vi "_Main_ByRuns_DAC2022_V1.0.2.vi"() -> ()   [LabVIEW 2017]
uses:
  <vilib>/Instr/_visa.llb/VISA Configure Serial Port (Instr).vi
panel:
  in  "Bias, kV/cm":dbl
  out "Field, kV/cm":dbl
  out "Current, mA":dbl
  out "Voltage, V":dbl
  in  "COM DAC":refnum<visa-resource-name>
  in  "WaveForm":i32(listbox)
  in  "Auto\nturn OFF":bool=TRUE
  in  "Content":i32(listbox)
  out "LastTrigTimer, s":dbl
  in  "Graph every, cycle":dbl=10.0 min=1.0 max=100.0
  in  "SendPeriod, ms":dbl=100.0 min=10.0 max=10000.0
  out "RunsNeed":i32
  out "Time LOG":cluster{dbl[], dbl[]}(graph)
  out "TrigTimer, s":dbl
  out "Bytes at Port":u32
  out "RecTry":i32
  out "OutVoltage, V":dbl
  in  "Exposition, s":dbl=3.0
  out "Channel 2, V":dbl format="%#_5g"
  out "Channel 1, V":dbl format="%#_5g"
  in  "Stop Button":bool
  in  "Start Button":bool
  in  "Sample H, um":dbl=32.0
  out "VoltageArray, V":dbl[](array[numeric])
  out "Shutter Red":bool
  out "Shutter Green":bool
  in  "Frames In Run":u32=180
  out "Global Frame Done":u32
  out "Now is Run #":u32
  out "Frame In Run Done":u32
  in  "Step, kV/cm":dbl=1.0 min=0.01 max=1000.0
  in  "Amplitude, kV/cm":dbl=10.0 min=10.0 max=1500.0
  in  "LOG file":path
  in  "COM ADC":refnum<visa-resource-name>
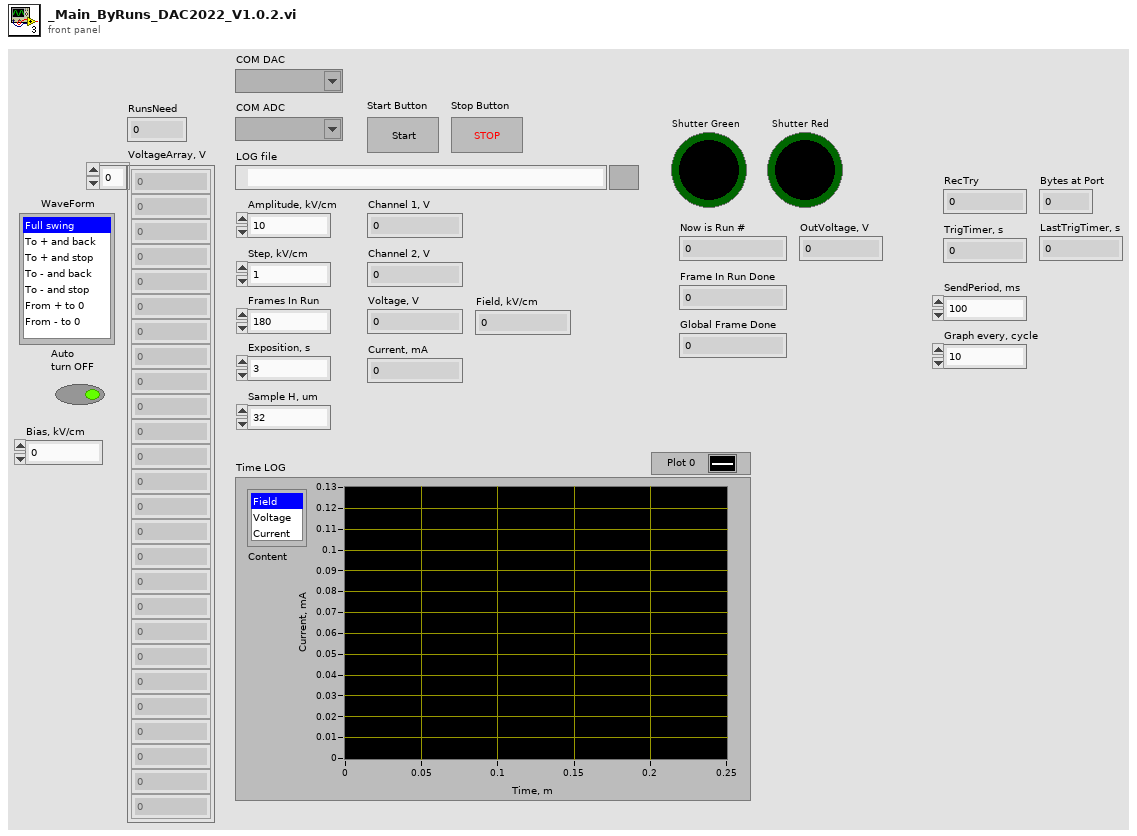
[diagram p1: front panel]
types:
  T1 = cluster{i32, i32, u32, "TrigState":bool, "TrigTimer, s":dbl, "CurrentError":bool}
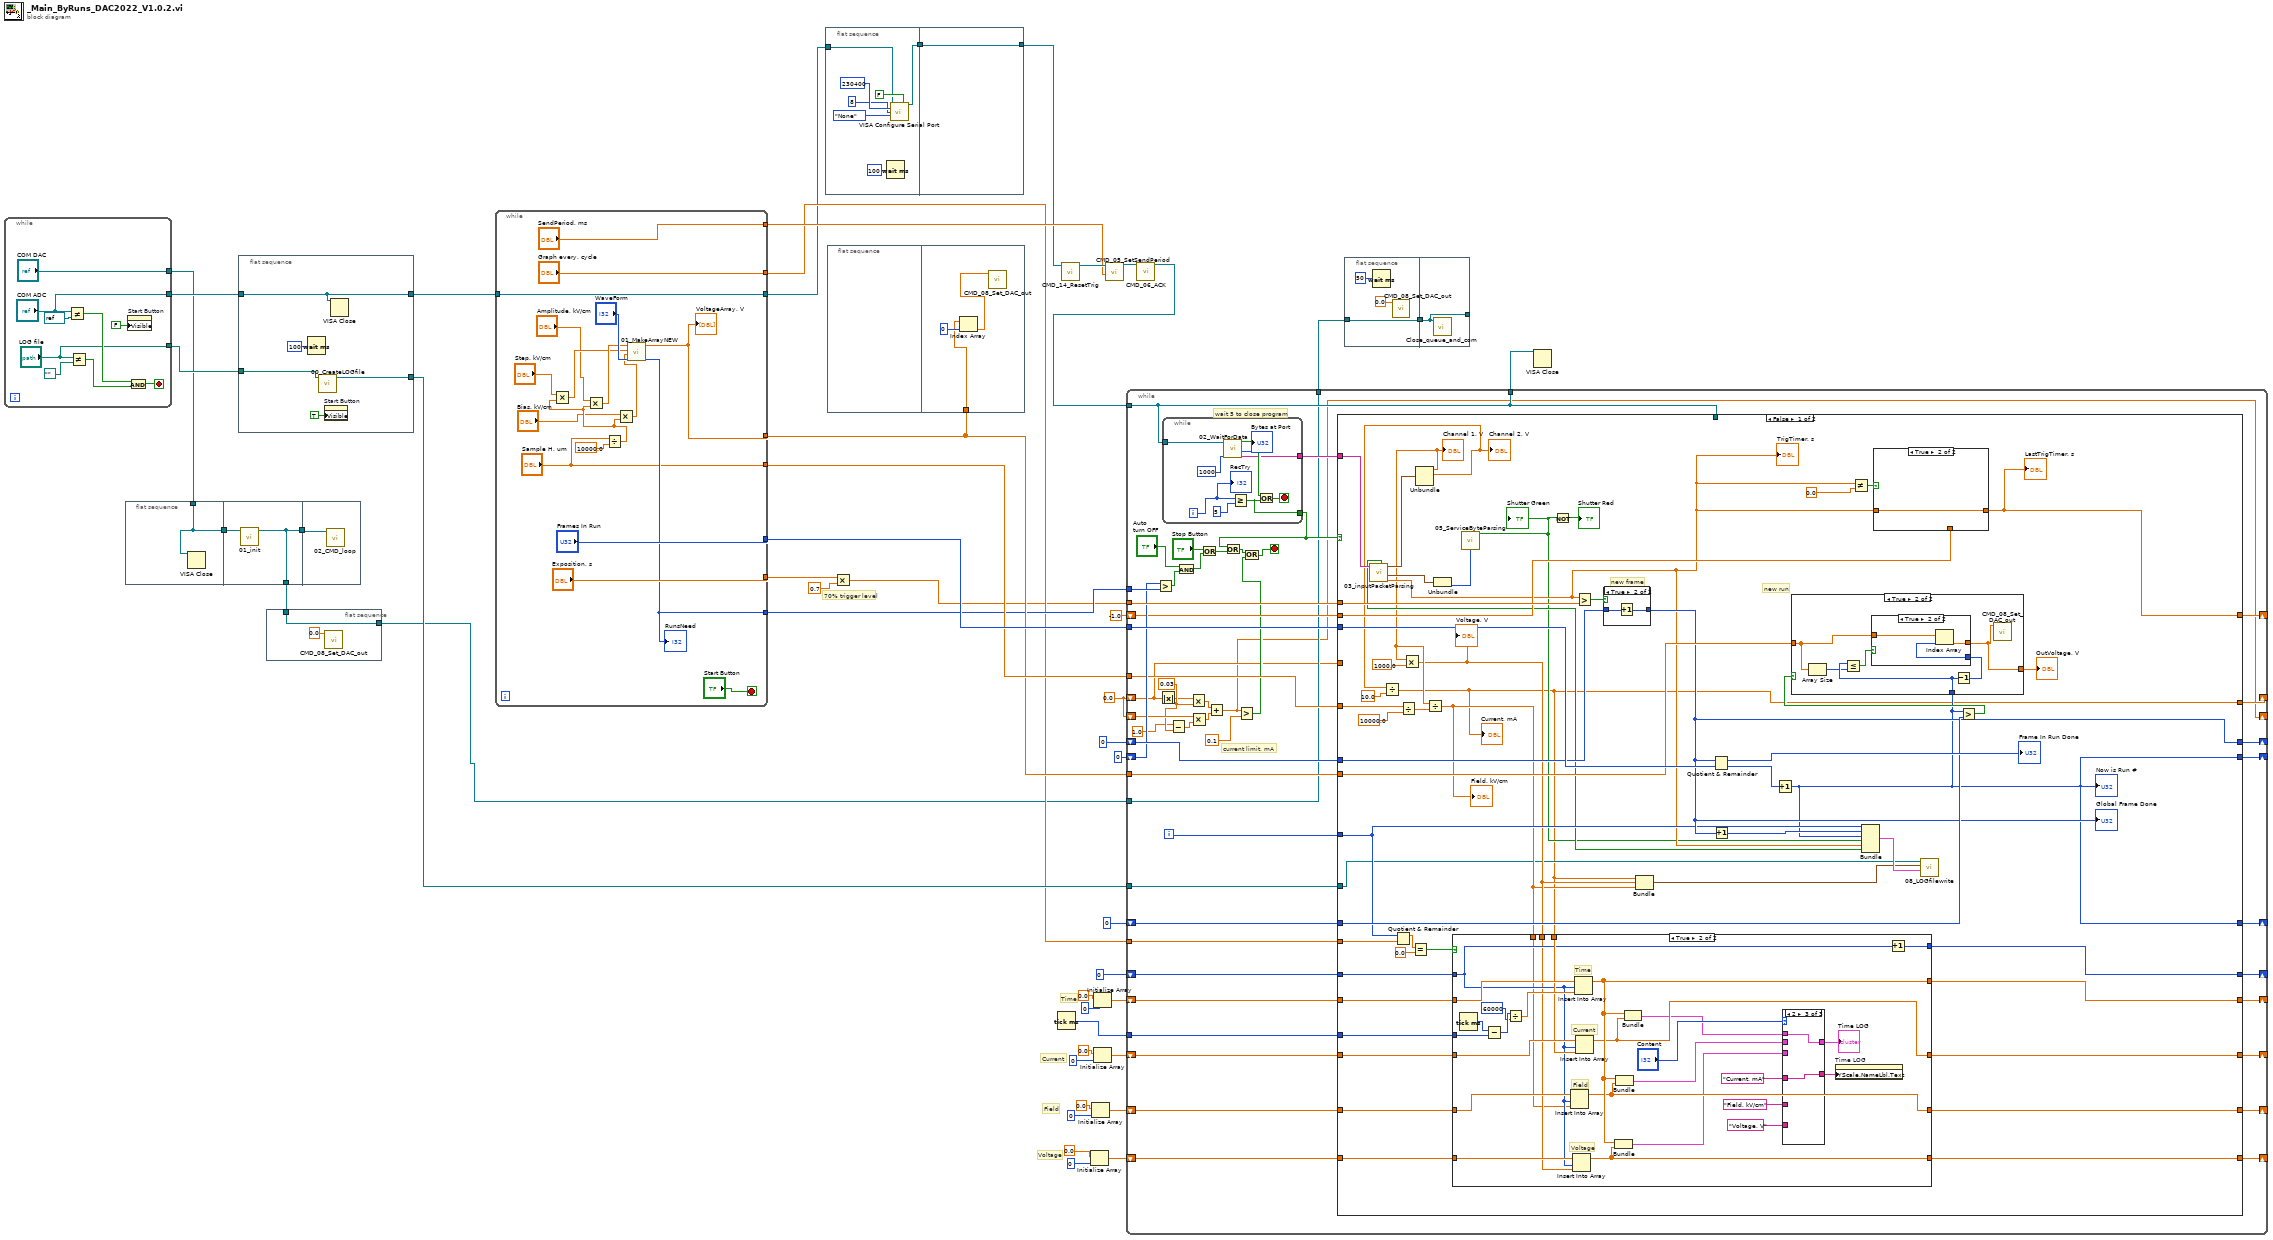
[diagram p0: block diagram]
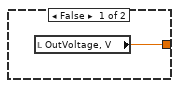
[diagram p6: hidden frame]
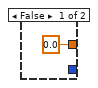
[diagram p7: hidden frame]
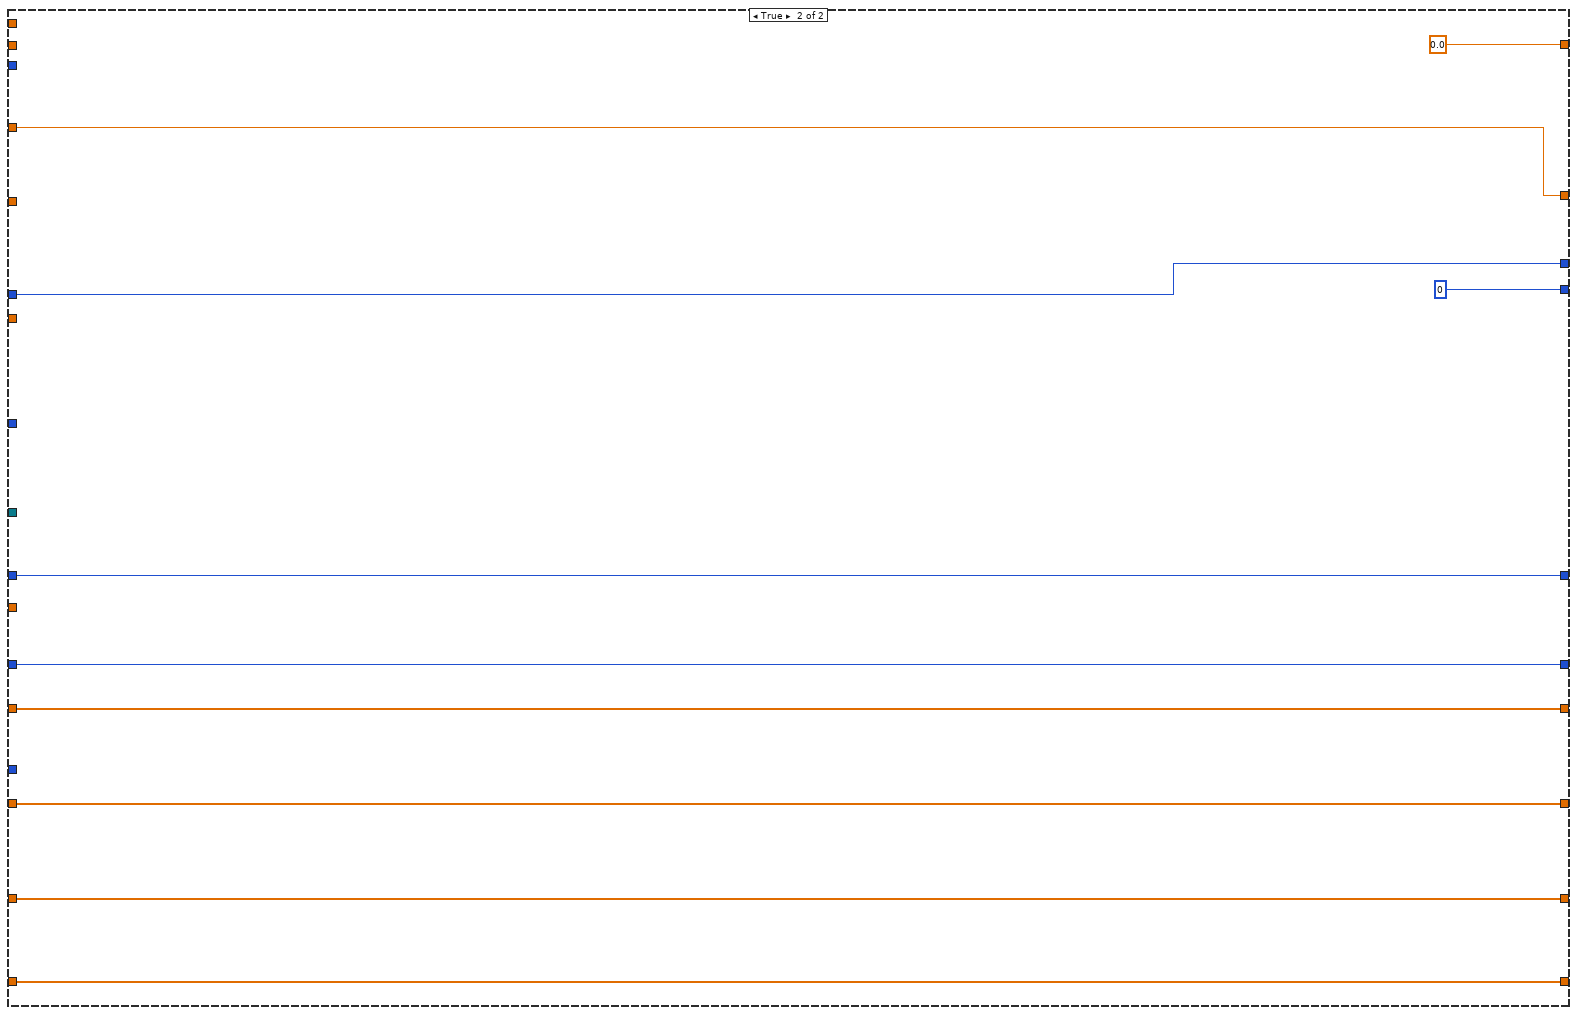
[diagram p9: hidden frame]
diagram:
  w1 = 0.0
  # "70% trigger level"
  # "Voltage"
  # "Field"
  # "Time"
  # "Current"
  n1 = while {
    tunnel: ["COM ADC"] -> w15
    tunnel: ["LOG file"] -> w14
    tunnel: ["COM DAC"] -> w6
    stop <- w53 stop-if-true
    n2 = Not Equal?(x="COM ADC", y=refnum<visa-resource-name> refnum ("COM port")) -> (x != y?=w50:bool)
    n3 = Not Equal?(x="LOG file", y=path "" ("LOG file")) -> (x != y?=w51:bool)
    n4 = property on="Start Button" class="Bool"("Visible"=FALSE) -> ()  [unwired: 2 in, 2 out]
    n5 = And(x=w50, y=w51) -> (x .and. y?=w53:bool)
  }
  n6 = flat-sequence {
    tunnel: [w56] -> w8
    tunnel: w6 -> [w56]
    tunnel: w8 -> [w58]
    tunnel: [w57] -> w5
    tunnel: [w57] -> w7
    tunnel: w7 -> [w59]
    frame #0 {
      n7 = VISA Close(VISA resource name=w56) -> ()  [unwired: 1 in, 1 out]
    }
    frame #1 {
      n8 = call "01_init.vi"("COM port"=w58) -> ("VISA resource name out"=w57:refnum<visa-resource-name>)  [unwired: 8 in, 2 out]
    }
    frame #2 {
      n9 = call "02_CMD_loop.vi"("VISA resource name"=w59) -> ()  [unwired: 11 in]
    }
  }
  n10 = flat-sequence {
    tunnel: [w64] -> w44
    tunnel: w15 -> [w60]
    tunnel: w14 -> [w61]
    tunnel: [w60] -> w13
    frame #0 {
      n11 = Wait (ms)(milliseconds to wait=u32 100) -> ()  [unwired: 1 out]
      n12 = call "00_CreateLOGfile.vi"("LOG file"=w61) -> ("refnum out"=w64:refnum<file>)  [unwired: 10 in]
      n13 = property on="Start Button" class="Bool"("Visible"=TRUE) -> ()  [unwired: 2 in, 2 out]
      n14 = VISA Close(VISA resource name=w60) -> ()  [unwired: 1 in, 1 out]
    }
  }
  n15 = flat-sequence {
    tunnel: w5 -> [w65]
    tunnel: [w65] -> w2
    frame #0 {
      n16 = call "CMD_08_Set_DAC_out.vi"("DAC voltage, V"=0.0) -> ()  [unwired: 11 in]
    }
  }
  n17 = while {
    tunnel: w13 -> [w78]
    tunnel: [w78] -> w11
    tunnel: [w77] -> w38
    tunnel: ["Sample H, um"] -> w45
    tunnel: ["Frames In Run"] -> w46
    tunnel: ["Exposition, s"] -> w24
    tunnel: [w76] -> w29
    tunnel: ["SendPeriod, ms"] -> w27
    tunnel: ["Graph every, cycle"] -> w26
    stop <- "Start Button" stop-if-true
    n18 = Divide(x="Sample H, um", y=10000.0) -> (x/y=w69:dbl)
    n19 = Multiply(x="Step, kV/cm", y=w69) -> (x*y=w72:dbl)
    n20 = Multiply(x="Amplitude, kV/cm", y=w69) -> (x*y=w73:dbl)
    n21 = Multiply(x="Bias, kV/cm", y=w69) -> (x*y=w67:dbl)
    n22 = call "01_MakeArrayNEW.vi"("Amp"=w73, "Step"=w72, "Bias"=w67, "WaveForm"="WaveForm") -> ("Array"=w77:dbl[], "ArraySize"=w76:i32)  [unwired: 5 in]
    "VoltageArray, V" <- w77
    "RunsNeed" <- w76
  }
  n23 = flat-sequence {
    tunnel: w11 -> [w87]
    tunnel: [w86] -> w12
    tunnel: w12 -> [w92]
    tunnel: [w92] -> w10
    frame #0 {
      n24 = Wait (ms)(milliseconds to wait=u32 100) -> ()  [unwired: 1 out]
      n25 = call-poly "VISA Configure Serial Port"("VISA resource name"=w87, "Enable Termination\nChar (T)"=FALSE ("Enable Termination\nChar (T)"), "baud rate (9600)"=u32 230400, "data bits (8)"=u16 8, "parity (0:none)"=enum16{"None", "Odd", "Even", "Mark", "Space"}."None") -> ("VISA resource name out"=w86:refnum<visa-resource-name>)  [unwired: 9 in, 1 out]
    }
    frame #1 {
    }
  }
  n26 = flat-sequence {
    tunnel: w38 -> [w94]
    frame #0 {
    }
    frame #1 {
      n27 = Index Array(array=w94, index=0) -> (element=w93:dbl)
      n28 = call "CMD_08_Set_DAC_out.vi"("DAC voltage, V"=w93) -> ()  [unwired: 11 in]
    }
  }
  n29 = Multiply(x=w24, y=0.7) -> (x*y=w25:dbl)
  n30 = Tick Count (ms)() -> (millisecond timer value=w33:u32)
  n31 = call "CMD_14_ResetTrig.vi"("VISA resource name"=w10) -> ("VISA resource name out"=w41:refnum<visa-resource-name>)  [unwired: 10 in]
  n32 = Initialize Array(0.0 ("element"), 0 ("dimension size")) -> (w16:dbl[])
  n33 = Initialize Array(0.0 ("element"), 0 ("dimension size")) -> (w17:dbl[])
  n34 = Initialize Array(0.0 ("element"), 0 ("dimension size")) -> (w30:dbl[])
  n35 = Initialize Array(0.0 ("element"), 0 ("dimension size")) -> (w34:dbl[])
  n36 = call "CMD_05_SetSendPeriod.vi"("Period, ms"=w27, "VISA resource name"=w41) -> ("VISA resource name out"=w40:refnum<visa-resource-name>)  [unwired: 9 in]
  n37 = call "CMD_06_ACK.vi"("VISA resource name"=w40) -> ("VISA resource name out"=w39:refnum<visa-resource-name>)  [unwired: 10 in]
  n38 = while {
    tunnel: w39 -> [w112]
    tunnel: w38 -> [w135]
    tunnel: w46 -> [w141]
    tunnel: w25 -> [w143]
    tunnel: w45 -> [w113]
    tunnel: w44 -> [w142]
    shift-right: [w138] -> _
    shift-left: 0 -> [w140]
    shift-right: [w137] -> _
    shift-left: u32 0 -> [w136]
    shift-right: [w133] -> _
    shift-left: 0 -> [w134]
    tunnel: w33 -> [w131]
    shift-right: [w129] -> _
    shift-left: w34 -> [w132]
    shift-right: [w128] -> _
    shift-left: w30 -> [w130]
    tunnel: w29 -> [w124]
    shift-right: [w126] -> _
    shift-left: u32 0 -> [w123]
    tunnel: w26 -> [w120]
    shift-right: [w119] -> _
    shift-left: -1.0 ("TrigTimer, s") -> [w118]
    shift-right: [w115] -> _
    shift-left: w17 -> [w117]
    shift-right: [w114] -> _
    shift-left: w16 -> [w116]
    tunnel: [w111] -> w3
    tunnel: [w112] -> w9
    tunnel: w2 -> [w111]
    shift-right: [w110] -> _
    shift-left: w1 -> [w105]
    shift-right: [w96] -> _
    shift-left: w1 -> [w104]
    i -> [w139]
    stop <- w108 stop-if-true
    w102 = 0.03
    # "current limit, mA"
    # "wait 5 to close program"
    n39 = Greater?(x=w123, y=w124) -> (0:w121:bool)
    n40 = Absolute Value(x=w105) -> (abs(x)=w97:dbl)
    n41 = while {
      tunnel: w112 -> [w264]
      tunnel: [w267] -> w145
      tunnel: [w268] -> w144
      i -> [w266]
      stop <- w270 stop-if-true
      n42 = call "02_WaitForData.vi"("WaitTimeoutMS"=u32 1000, "VISA"=w264) -> ("Buffer"=w268:string, "Bytes at Port"=→"Bytes at Port":u32, "Data Recived"=w269:bool)  [unwired: 7 in]
      n43 = Greater Or Equal?(x=w266, y=5) -> (x >= y?=w267:bool)
      n44 = Or(x=w269, y=w267) -> (x .or. y?=w270:bool)
      "RecTry" <- w266
    }
    n45 = Subtract(x=1.0, y=w102) -> (x-y=w103:dbl)
    n46 = And(x="Auto\nturn OFF", y=w121) -> (x .and. y?=w122:bool)
    n47 = Multiply(x=w97, y=w102) -> (x*y=w99:dbl)
    n48 = Multiply(x=w104, y=w103) -> (x*y=w100:dbl)
    n49 = Or(x="Stop Button", y=w122) -> (x .or. y?=w127:bool)
    n50 = Add(x=w99, y=w100) -> (x+y=w96:dbl)
    n51 = Or(x=w145, y=w127) -> (x .or. y?=w107:bool)
    n52 = Greater?(x=w96, y=0.1) -> (0:w106:bool)
    n53 = Or(x=w107, y=w106) -> (x .or. y?=w108:bool)
    n54 = case shown="False" w145 {
      tunnel: w144 -> [w199 _]
      tunnel: w143 -> [w195 _]
      tunnel: w142 -> [w147 _]
      tunnel: w141 -> [w196 _]
      tunnel: w140 -> [w193 w263]
      tunnel: w139 -> [w180 _]
      tunnel: [w185 w263] -> w138
      tunnel: [w171 w262] -> w137
      tunnel: w136 -> [w188 w262]
      tunnel: w135 -> [w189 _]
      tunnel: w112 -> [_ _]
      tunnel: w134 -> [w178 w261]
      tunnel: [w177 w261] -> w133
      tunnel: w132 -> [w176 w260]
      tunnel: w131 -> [w175 _]
      tunnel: w130 -> [w174 w259]
      tunnel: [w173 w260] -> w129
      tunnel: [w172 w259] -> w128
      tunnel: [w171 u32 0] -> w126
      tunnel: w120 -> [w170 _]
      tunnel: [w167 0.0 ("TrigTimer, s")] -> w119
      tunnel: w118 -> [w166 _]
      tunnel: w117 -> [w162 w256]
      tunnel: w116 -> [w161 w255]
      tunnel: [w160 w256] -> w115
      tunnel: [w159 w255] -> w114
      tunnel: w113 -> [w153 _]
      tunnel: [w146 w254] -> w110
      tunnel: w105 -> [_ w254]
      frame False {
        # "new run"
        # "new frame"
        n55 = call "03_inputPacketParsing.vi"("string"=w199) -> ("TrigTimer, s"=w165:dbl, "Service state"=w184:cluster{u8, u8}, "Voltage"=w197:cluster{dbl, dbl, dbl, dbl}, "CurrentError"=w164:bool)  [unwired: 6 in, 1 out]
        "TrigTimer, s" <- w165
        n56 = Quotient & Remainder(x=w180, y=w170) -> (x-y*floor(x/y)=w182:dbl)  [unwired: 1 out]
        n57 = Divide(x=w153, y=10000.0) -> (x/y=w154:dbl)
        n58 = Equal?(x=w182, y=0.0) -> (x = y?=w179:bool)
        n59 = Unbundle(w197) -> (w155:dbl, w157:dbl)  [unwired: 2 out]
        "Channel 1, V" <- w155
        "Channel 2, V" <- w157
        n60 = Divide(x=w157, y=10.0) -> (x/y=w146:dbl)
        "Current, mA" <- w146
        n61 = Multiply(x=w155, y=1000.0) -> (x*y=w150:dbl)
        "Voltage, V" <- w150
        n62 = Divide(x=w155, y=w154) -> (x/y=w149:dbl)
        "Field, kV/cm" <- w149
        n63 = Unbundle(w184) -> (w183:u8)  [unwired: 1 out]
        n64 = case shown="True" w179 {
          tunnel: w178 -> [w206 w222]
          tunnel: [w206 w229] -> w177
          tunnel: w176 -> [w204 w227]
          tunnel: w175 -> [_ w232]
          tunnel: w174 -> [w205 w226]
          tunnel: [w205 w218] -> w172
          tunnel: [w204 w221] -> w173
          tunnel: w146 -> [_ w225]
          tunnel: w162 -> [w203 w224]
          tunnel: w161 -> [w202 w223]
          tunnel: [w203 w219] -> w160
          tunnel: [w202 w220] -> w159
          tunnel: w150 -> [_ w208]
          tunnel: w149 -> [_ w207]
          frame False {
          }
          frame True {
            # "Time"
            # "Voltage"
            # "Field"
            # "Current"
            n65 = Tick Count (ms)() -> (millisecond timer value=w233:u32)
            n66 = Subtract(x=w233, y=w232) -> (x-y=w231:u32)
            n67 = Divide(x=w231, y=u32 60000) -> (x/y=w228:dbl)
            n68 = Insert Into Array(array=w224, index=w222, new element=w207) -> (w219:dbl[])
            n69 = Insert Into Array(array=w223, index=w222, new element=w208) -> (w220:dbl[])
            n70 = Insert Into Array(array=w227, index=w222, new element=w228) -> (w221:dbl[])
            n71 = Insert Into Array(array=w226, index=w222, new element=w225) -> (w218:dbl[])
            n72 = Bundle(w221, w220) -> (w214:cluster{dbl[], dbl[]})  [unwired: 1 in]
            n73 = Bundle(w221, w219) -> (w215:cluster{dbl[], dbl[]})  [unwired: 1 in]
            n74 = Bundle(w221, w218) -> (w216:cluster{dbl[], dbl[]})  [unwired: 1 in]
            n75 = case shown="2" "Content" {
              tunnel: w216 -> [_ _ w239]
              tunnel: w215 -> [w235 _ _]
              tunnel: w214 -> [_ w237 _]
              tunnel: [w235 w237 w239] -> w213
              tunnel: "Current, mA" ("Y Scale.Name Label.Text") -> [_ _ w238]
              tunnel: "Field, kV/cm" ("Y Scale.Name Label.Text") -> [w234 _ _]
              tunnel: "Voltage, V" ("Y Scale.Name Label.Text") -> [_ w236 _]
              tunnel: [w234 w236 w238] -> w209
              frame 0, Default {
              }
              frame 1 {
              }
              frame 2 {
              }
            }
            "Time LOG" <- w213
            n76 = property on="Time LOG" class="XYGraph (strict)"("YScale.NameLbl.Text"=w209) -> ()  [unwired: 2 in, 2 out]
            n77 = Increment(x=w222) -> (x+1=w229:i32)
          }
        }
        n78 = call "05_ServiceByteParsing.vi"("InputByte"=w183) -> ("TrigState"=w163:bool)  [unwired: 7 in, 3 out]
        "Shutter Green" <- w163
        n79 = Not(x=w163) -> (.not. x?=→"Shutter Red":bool)
        n80 = Greater?(x=w165, y=w195) -> (0:w194:bool)
        n81 = case shown="True" w194 {
          tunnel: w193 -> [w251 w253]
          tunnel: [w251 w252] -> w185
          frame False {
          }
          frame True {
            n82 = Increment(x=w253) -> (x+1=w252:i32)
          }
        }
        "Global Frame Done" <- w185
        n83 = Bundle(w146, w150, w149) -> (w148:cluster{dbl, dbl, dbl})  [unwired: 1 in]
        n84 = Quotient & Remainder(x=w185, y=w196) -> (x-y*floor(x/y)=→"Frame In Run Done":u32, floor(x/y)=w191:u32)
        n85 = Increment(x=w185) -> (x+1=w186:i32)
        n86 = Increment(x=w191) -> (x+1=w171:u32)
        "Now is Run #" <- w171
        n87 = Not Equal?(x=w165, y=0.0) -> (x != y?=w169:bool)
        n88 = Bundle(w180, w186, w171, "TrigState"=w163, "TrigTimer, s"=w165, "CurrentError"=w164) -> (w151:T1)  [unwired: 1 in]
        n89 = case shown="True" w169 {
          tunnel: [w200 w201] -> w167
          tunnel: w165 -> [_ w201]
          tunnel: w166 -> [w200 _]
          frame False {
          }
          frame True {
          }
        }
        "LastTrigTimer, s" <- w167
        n90 = call "08_LOGfilewrite.vi"("Counters"=w151, "output cluster"=w148, "refnum out"=w147) -> ()  [unwired: 9 in]
        n91 = Greater?(x=w171, y=w188) -> (0:w192:bool)
        n92 = case shown="True" w192 {
          tunnel: w189 -> [_ w242]
          tunnel: w171 -> [_ w245]
          tunnel: [w240 w241] -> w187
          frame False {
            n93 = local read "OutVoltage, V"() -> (w240:dbl)
          }
          frame True {
            n94 = Array Size(array=w242) -> (size(s)=w244:i32)
            n95 = Less Or Equal?(x=w245, y=w244) -> (x <= y?=w243:bool)
            n96 = Decrement(x=w245) -> (x-1=w246:u32)
            n97 = case shown="True" w243 {
              tunnel: w246 -> [_ w250]
              tunnel: w242 -> [_ w249]
              tunnel: [0.0 w248] -> w241
              frame False {
              }
              frame True {
                n98 = Index Array(array=w249, index=w250) -> (element=w248:dbl)
              }
            }
            n99 = call "CMD_08_Set_DAC_out.vi"("DAC voltage, V"=w241) -> ()  [unwired: 11 in]
          }
        }
        "OutVoltage, V" <- w187
      }
      frame True {
      }
    }
  }
  n100 = flat-sequence {
    tunnel: w3 -> [w274]
    tunnel: [w274] -> w4
    tunnel: [w276] -> _
    tunnel: w4 -> [w276]
    frame #0 {
      n101 = Wait (ms)(milliseconds to wait=u32 50) -> ()  [unwired: 1 out]
      n102 = call "CMD_08_Set_DAC_out.vi"("DAC voltage, V"=0.0) -> ()  [unwired: 11 in]
    }
    frame #1 {
      n103 = call "Close_queue_and_com.vi"("VISA"=w276) -> ()  [unwired: 11 in]
    }
  }
  n104 = VISA Close(VISA resource name=w9) -> ()  [unwired: 1 in, 1 out]
